vi "Project New.vi"(8 "error in":errorcluster) -> (0 "error out":errorcluster caption="错误输出")   [LabVIEW 2016]
uses:
  DAQ-VirtualCH/SubVIs/VCH/Private/Ctrls/PSVCH_VCH Info.ctl
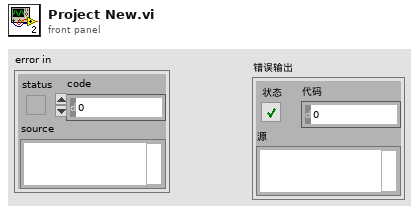
[diagram p1: front panel]
types:
  T1 = typedef "PSVCH_VCH Info.ctl" = cluster{"Tag":string[], "Tag String":string[], "Name":string[], "Enable":bool[], "Formula":string[], "Unit":string[], "Save":bool[], "Time":i64[]}
  T2 = cluster{"TREE PNG":path, "User Guide":path, "DefaultSave":path, "BuildPath":path, "Image":path, "Modules":path, "Configuration":path, "License":path, "SplitFiles":path, "System.ini":path}
  T3 = typedef "Global para Config.ctl" = cluster{"连续存储设置":cluster{"Save Mode":i32, "Sel Save Mode":i32, "FolderPath":path, "Filename":string, "Explation":string, "AutoPoint":i32, "Template":path}, "Latest Prj":path, "Tdms Ref*":refnum<k34>, "默认波形图个数":u8, "列表列数":u8}
  T4 = enum16{"Run", "Pause", "Stop", "DAQ Chl", "Save", "Update Data", "Symbol Path", "DAQ DATA Queues", "None"}
  T5 = cluster{"Main Queue":string, "DAQ Queue":string, "ANA Queue":string, "CUI Queue":string, "Q-FocusList":string, "Q-Toolbar":string, "Q-Config":string}
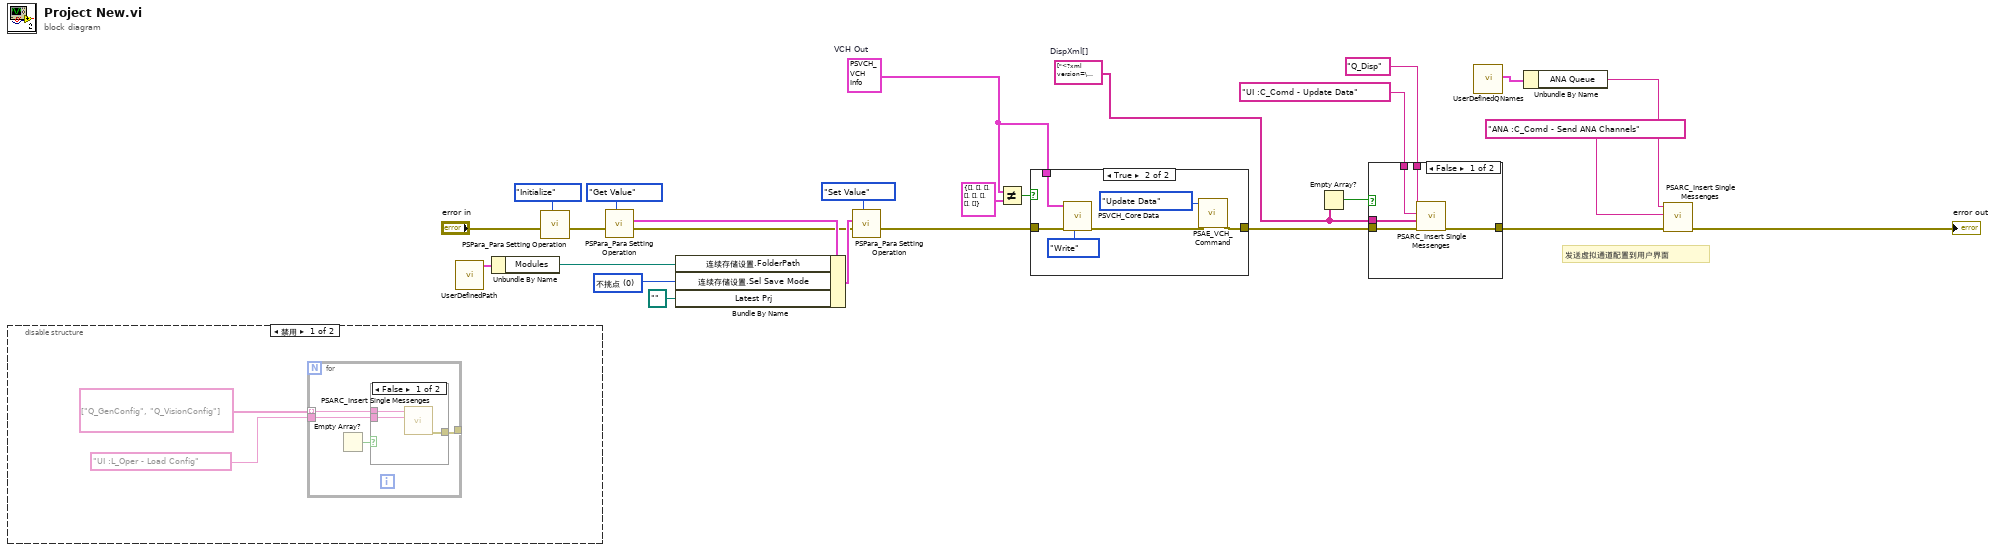
[diagram p0: block diagram]
diagram:
  w6 = 0 items=["不挑点", "自动挑点", "手动挑点"] ("Save Mode")
  w16 = string[] ["<?xml version=\"1.0\" encoding=\"UTF-8\" standalone=\"no\" ?><Root InsertViPath=\"..\\..\\Team-Library\\ApplicationLib\\X-DAQ Viewer\\SubVIs\\New_GraphDispWithTime.vi\" InsertViValue=\"&lt;Cluster>\r&#xA;&lt;Name>ViValue&lt;/Name>\r&#xA;&lt;NumElts>5&lt;/NumElts>\r&#xA;&lt;String>\r&#xA;&lt;Name>CHTag&lt;/Name>\r&#xA;&lt;Val>&lt;/Val>\r&#xA;&lt;/String>\r&#xA;&lt;Cluster>\r&#xA;&lt;Name>GraphProperts&lt;/Name>\r&#xA;&lt;NumElts>3&lt;/NumElts>\r&#xA;&lt;DBL>\r&#xA;&lt;Name>YMax&lt;/Name>\r&#xA;&lt;Val>10.00000000000000&lt;/Val>\r&#xA;&lt;/DBL>\r&#xA;&lt;DBL>\r&#xA;&lt;Name>YMin&lt;/Name>\r&#xA;&lt;Val>0.00000000000000&lt;/Val>\r&#xA;&lt;/DBL>\r&#xA;&lt;U8>\r&#xA;&lt;Name>ScaleFit&lt;/Name>\r&#xA;&lt;Val>2&lt;/Val>\r&#xA;&lt;/U8>\r&#xA;&lt;/Cluster>\r&#xA;&lt;String>\r&#xA;&lt;Name>CHUnit&lt;/Name>\r&#xA;&lt;Val>&lt;/Val>\r&#xA;&lt;/String>\r&#xA;&lt;String>\r&#xA;&lt;Name>CHName&lt;/Name>\r&#xA;&lt;Val>&lt;/Val>\r&#xA;&lt;/String>\r&#xA;&lt;String>\r&#xA;&lt;Name>CHValue&lt;/Name>\r&#xA;&lt;Val>-----&lt;/Val>\r&#xA;&lt;/String>\r&#xA;&lt;/Cluster>\r&#xA;\" SplitMode=\"-1\"/>"]  # DispXml[]
  w17 = T1 {"Tag"=["VCH1", "VCH2", "VCH3", "VCH4", "VCH5", "VCH6", "VCH7", "VCH8"], "Tag String"=["VCH1", "VCH2", "VCH3", "VCH4", "VCH5", "VCH6", "VCH7", "VCH8"], "Name"=["VCH1", "VCH2", "VCH3", "VCH4", "VCH5", "VCH6", "VCH7", "VCH8"], "Enable"=[FALSE, FALSE, FALSE, FALSE, FALSE, FALSE, FALSE, FALSE], "Formula"=["", "", "", "", "", "", "", ""], "Unit"=["V", "V", "V", "V", "V", "V", "V", "V"], "Save"=[TRUE, TRUE, TRUE, TRUE, TRUE, TRUE, TRUE, TRUE], "Time"=[1000, 1000, 1000, 1000, 1000, 1000, 1000, 1000]}  # VCH Out
  # "发送虚拟通道配置到用户界面"
  n1 = disable-structure shown="禁用" {
    frame Disabled {
      n2 = for {
        tunnel: string[] ["Q_GenConfig", "Q_VisionConfig"] -> [w32] mode=indexing
        tunnel: "UI :L_Oper - Load Config" -> [w31]
        tunnel: [w30] -> _
        n3 = Empty Array?() -> (empty?=w29:bool)  [unwired: 1 in]
        n4 = case shown="False" w29 {
          tunnel: w32 -> [w35 _]
          tunnel: w31 -> [w34 _]
          tunnel: [w33 _] -> w30
          frame False {
            n5 = call <vilib>:"PSARC_Insert Single Messenges.vi"("Order"=w34, "Queue Name"=w35) -> ("error out"=w33:errorcluster)  [unwired: 9 in]
          }
          frame True {
          }
        }
      }
    }
    frame Enabled {
    }
  }
  n6 = call "UserDefinedPath.vi"() -> ("UserDefinedPath"=w8:T2)  [unwired: 11 in]
  n7 = Unbundle By Name(w8) -> ("Modules"=w7:path)
  n8 = call "PSPara_Para Setting Operation.vi"("Operation"=enum16{"Set Value", "Get Value", "Initialize"}."Initialize", "error in (no error)"="error in") -> ("error out"=w12:errorcluster)  [unwired: 8 in, 1 out]
  n9 = call "PSPara_Para Setting Operation.vi"("Operation"=enum16{"Set Value", "Get Value", "Initialize"}."Get Value", "error in (no error)"=w12) -> ("error out"=w9:errorcluster, "_Para"=w11:T3)  [unwired: 8 in]
  n10 = Bundle By Name(cluster=w11, "连续存储设置.FolderPath"=w7, "连续存储设置.Sel Save Mode"=w6, "Latest Prj"=path "" ("ConfigDS Path*")) -> (w13:T3)
  n11 = call "PSPara_Para Setting Operation.vi"("Operation"=enum16{"Set Value", "Get Value", "Initialize"}."Set Value", "error in (no error)"=w9, "_Para"=w13) -> ("error out"=w4:errorcluster)  [unwired: 7 in, 1 out]
  n12 = Not Equal?(x=w17, y=T1 {"Tag"=[], "Tag String"=[], "Name"=[], "Enable"=[], "Formula"=[], "Unit"=[], "Save"=[], "Time"=[]}) -> (x != y?=w19:bool)
  n13 = case shown="True" w19 {
    tunnel: w4 -> [w36 w41]
    tunnel: [w36 w38] -> w24
    tunnel: w17 -> [_ w37]
    frame False {
    }
    frame True {
      n14 = call "PSVCH_Core Data.vi"("Oper"=enum16{"Init", "Read", "Write"}."Write", "Error In (no error)"=w41, "VCH In"=w37) -> ("Error Out"=w39:errorcluster)  [unwired: 7 in, 1 out]
      n15 = call "PSAE_VCH_Command.vi"("Error In (no error)"=w39, "Comd"=T4."Update Data") -> ("Error Out"=w38:errorcluster)  [unwired: 9 in]
    }
  }
  n16 = Empty Array?(array=w16) -> (empty?=w18:bool)
  n17 = case shown="False" w18 {
    tunnel: "Q_Disp" ("Queue Name(unamed)") -> [w47 _]
    tunnel: "UI :C_Comd - Update Data" ("Queue Name(unamed)") -> [w46 _]
    tunnel: w24 -> [w45 w48]
    tunnel: [w44 w48] -> w23
    tunnel: w16 -> [w43 _]
    frame False {
      n18 = call <vilib>:"PSARC_Insert Single Messenges.vi"("error in (no error)"=w45, "Data"=w43, "Order"=w46, "Queue Name"=w47) -> ("error out"=w44:errorcluster)  [unwired: 7 in]
    }
    frame True {
    }
  }
  n19 = call "UserDefinedQNames.vi"() -> ("All Queues"=w1:T5)  [unwired: 11 in]
  n20 = Unbundle By Name(w1) -> ("ANA Queue"=w21:string)
  n21 = call <vilib>:"PSARC_Insert Single Messenges.vi"("error in (no error)"=w23, "Order"="ANA :C_Comd - Send ANA Channels", "Queue Name"=w21) -> ("error out"=→"error out":errorcluster)  [unwired: 8 in]
